vi "UHR-Fleezers Control (host) -TL - oscillation.vi"(0 "Tab Control":T5(tab)) -> ()   [LabVIEW 2013] (continued)
            n1087 = flat-sequence {
              tunnel: w1684 -> [w1698]
              tunnel: w1685 -> [w1694]
              tunnel: w1683 -> [_]
              tunnel: w1685 -> [w1700]
              tunnel: w1684 -> [w1701]
              frame #0 {
                n1088 = local read "All Pump Parameters"() -> (w1693:T6)
                n1089 = Multiply(x=60.0, y="Flush Center Ch Rate (ul/m)") -> (x*y=w1690:dbl)
                n1090 = Unbundle By Name(w1693) -> ("Pump 2"=w1699:T32)
                n1091 = call "Set pump parameters.vi"("Pump write delay (ms)"=w1694, "Volume (uL)"="Flush Center Ch Volume (uL)", "Rate (uL/h)"=w1690, "Units"=3.0, "Pump #"=2.0, "Pump Parameters In"=w1699, "VISA resource name"=w1698) -> ("Pump Parameters Out"=w1692:T32)  [unwired: 3 in]
                n1092 = Bundle By Name(cluster=w1693, "Pump 2"=w1692) -> (w1691:T6)
                n1093 = local write "All Pump Parameters"(w1691) -> ()
                n1094 = Add(x="Flush Center Ch Volume (uL)", y="Total Volume\nFlushed (uL)") -> (x+y=w1687:dbl)
                n1095 = local write "Total Volume\nFlushed (uL)"(w1687) -> ()
              }
              frame #1 {
                n1096 = Wait (ms)(milliseconds to wait=w1700) -> ()  [unwired: 1 out]
              }
              frame #2 {
                n1097 = call "Write to pump.vi"("string"="start", "VISA resource name"=w1701) -> ()  [unwired: 1 out]
              }
            }
            n1098 = local read "Chemyx Syringe Pump Serial Port"() -> (w1684:refnum<visa-resource-name>)
          }
          frame Enabled {
            n1099 = call "hamilton_controller.vi"("Open?"=w1703, "valve"=enum16{"A", "B", "C", "D", "ALL"}."B", "action"=T20."MOVE VALVE") -> ()  [unwired: 8 in, 1 out]
          }
        }
      }
      event "Main:": Value Change {
        n1100 = event-data() -> ()  [unwired: 7 out]
        n1101 = call "hamilton_controller.vi"("Open?"="Main:", "valve"=enum16{"A", "B", "C", "D", "ALL"}."C", "action"=T20."MOVE VALVE") -> ()  [unwired: 8 in, 1 out]
      }
      event "Shunt:": Value Change {
        n1102 = event-data() -> ()  [unwired: 7 out]
        n1103 = call "hamilton_controller.vi"("Open?"="Shunt:", "valve"=enum16{"A", "B", "C", "D", "ALL"}."D", "action"=T20."MOVE VALVE") -> ()  [unwired: 8 in, 1 out]
      }
      event "Flip Green Filter": Value Change {
        n1104 = event-data() -> ()  [unwired: 7 out]
        n1105 = local write "Flip Green Filter"("Flip Green Filter") -> ()
        n1106 = flat-sequence {
          tunnel: w1719 -> [w1724]
          tunnel: w1718 -> [w1723]
          tunnel: [w1721] -> w1716
          tunnel: [w1720] -> w1715
          tunnel: [w1726] -> w1714
          tunnel: w1716 -> [w1726]
          tunnel: [w1725] -> w1713
          tunnel: w1715 -> [w1725]
          tunnel: w1714 -> [w1730]
          tunnel: w1713 -> [w1729]
          tunnel: [w1728] -> w1717
          frame #0 {
            n1107 = xnode "Read/Write Control"("FPGA VI Reference In"=w1724, "error in"=w1723, "Green Filter Flipper"=TRUE) -> ("FPGA VI Reference Out"=w1721:T19, "error out"=w1720:errorcluster)
          }
          frame #1 {
            n1108 = Wait (ms)(milliseconds to wait=u32 100) -> ()  [unwired: 1 out]
          }
          frame #2 {
            n1109 = xnode "Read/Write Control"("FPGA VI Reference In"=w1730, "error in"=w1729, "Green Filter Flipper"=FALSE) -> ("error out"=w1728:errorcluster)  [unwired: 1 out]
          }
        }
      }
      event "Pump 1 contents", "Pump 3 contents": Value Change {
        n1110 = event-data() -> ()  [unwired: 7 out]
        n1111 = local read "Pump 1 contents"() -> (→"Pump 1 cont disp":string)
        n1112 = local read "Pump 3 contents"() -> (→"Pump 3 cont disp":string)
      }
      event "Reset Trap Pos. FB": Value Change {
        n1113 = event-data() -> ()  [unwired: 7 out]
        n1114 = xnode "Read/Write Control"("FPGA VI Reference In"=w1736, "error in"=w1735, "Trap Pos. FB Reset"="Reset Trap Pos. FB") -> ()  [unwired: 2 out]
      }
      event "Trap Pos. FB ON": Value Change {
        n1115 = event-data() -> ()  [unwired: 7 out]
        n1116 = xnode "Read/Write Control"("FPGA VI Reference In"=w1739, "error in"=w1738, "Force feedback"="Trap Pos. FB ON") -> ()  [unwired: 2 out]
      }
      event "Trap Pos. FB Range", "Trap Pos. FB Gains", "Trap Pos. FB Mult Factor", "Trap Pos. FB Offset Factor", "Trap Pos FB Negate Action", "Trap Pos FB Monitor\nT1 or T2": Value Change {
        n1117 = event-data() -> ()  [unwired: 7 out]
        n1118 = xnode "Read/Write Control"("FPGA VI Reference In"=w1748, "error in"=w1747, "Trap Pos. FB Range"="Trap Pos. FB Range", "Trap Pos. FB Gains"="Trap Pos. FB Gains", "Trap Pos. FB Mult Factor"="Trap Pos. FB Mult Factor", "Trap Pos. FB Offset Factor"="Trap Pos. FB Offset Factor", "Trap Pos FB Negate Action"="Trap Pos FB Negate Action", "Trap Pos FB Monitor T1 or T2"="Trap Pos FB Monitor\nT1 or T2", "AI1 X Scale"="Trap Pos. AI1 X Pre-scale") -> ()  [unwired: 2 out]
      }
      event "Trap Pos FB SP": Value Change {
        n1119 = event-data() -> ()  [unwired: 7 out]
        n1120 = xnode "Read/Write Control"("FPGA VI Reference In"=w1751, "error in"=w1750, "Trap Pos. FB SP"="Trap Pos FB SP") -> ()  [unwired: 2 out]
      }
      event "Set SP to Reading": Value Change {
        n1121 = event-data() -> ()  [unwired: 7 out]
        n1122 = local read "Trap Pos FB Monitor\nT1 or T2"() -> (w1759:bool)
        n1123 = local read "Trap X AI1 (DMA)"() -> (w1762:T13)
        n1124 = local read "Trap X (AI1)"() -> (w1765:T1)
        n1125 = Unbundle By Name(w1765) -> ("Trap 1"=w1764:fxp<+/-,16,1>, "Trap 2"=w1763:fxp<+/-,16,1>)
        n1126 = Unbundle By Name(w1762) -> ("Set 1"=w1761:fxp<+/-,16,1>, "Set 2"=w1760:fxp<+/-,16,1>)
        n1127 = Select(t=w1764, s=w1759, f=w1763) -> (s? t:f=w1758:fxp<+/-,16,1>)
        n1128 = Select(t=w1761, s=w1759, f=w1760) -> (s? t:f=w1757:fxp<+/-,16,1>)
        n1129 = Not(x="Set SP Using...") -> (.not. x?=w1752:bool)
        n1130 = Select(t=w1758, s=w1752, f=w1757) -> (s? t:f=w1753:fxp<+/-,16,1>)
        n1131 = xnode "Read/Write Control"("FPGA VI Reference In"=w1755, "error in"=w1754, "Trap Pos. FB SP"=w1753) -> ()  [unwired: 2 out]
        n1132 = local write "Trap Pos FB SP"(w1753) -> ()
      }
      event "Trap Pos. FB Out Scale 2^n": Value Change {
        n1133 = event-data() -> ()  [unwired: 7 out]
        n1134 = Scale By Power Of 2(n="Trap Pos. FB Out Scale 2^n", x=ext 1.0) -> (x*2^n=w1767:ext)
        n1135 = property on="Trap Pos. FB Mult Factor" class="DigNum (strict)"("Val(Sgnl)"=w1767) -> ()  [unwired: 2 in, 2 out]
      }
      event "Trap Pos FB Int Count": Value Change {
        n1136 = event-data() -> ()  [unwired: 7 out]
        n1137 = xnode "Read/Write Control"("FPGA VI Reference In"=w1772, "error in"=w1771, "Trap Pos FB Int Count"="Trap Pos FB Int Count") -> ()  [unwired: 2 out]
      }
    }
    "error out 2" <- w950
    n1138 = node-c288() -> ()  [unwired: 1 in, 1 out]
  }
  n1139 = node-c288() -> (w79:T24)  [unwired: 4 out]
  n1140 = timed-loop "Mouse control: trap position (AOM deflection), set confocal spot from image" {
    tunnel: [w1774] -> w38
    tunnel: w2 -> [w1773]
    timing: w79 -> [_]
    timing-out: [_] -> w78
    stop <- w1774 stop-if-true
    n1141 = node-c288() -> ()  [unwired: 2 out]
    n1142 = event shown="[0] \"Pane\": Mouse Down" {
      selector: _ -> [_ _]
      dyn-events: _ -> [_ _]
      timeout: _ -> [_ _]
      tunnel: w1773 -> [w1777 _]
      event Mouse Down {
        n1143 = event-data() -> ("Time"=w1779:u32, "Coords"=w1778:T8, "Button"=w1780:u16)  [unwired: 6 out]
        n1144 = case shown="1" w1780 {
          tunnel: w1779 -> [_ _ w1883]
          tunnel: w1778 -> [_ w1817 w1881]
          tunnel: w1777 -> [_ _ w1879]
          frame 0, Default {
          }
          frame 1 {
            n1145 = property on="APD 2" class="ImageControl"() -> ("Displayed Image Position"=w1787:cluster{"Left":i32, "Top":i32})  [unwired: 2 in, 2 out]
            n1146 = property on="APD 1" class="ImageControl"() -> ("Displayed Image Position"=w1816:cluster{"Left":i32, "Top":i32})  [unwired: 2 in, 2 out]
            n1147 = property on="Detection Laser X" class="ImageControl"() -> ("Displayed Image Position"=w1813:cluster{"Left":i32, "Top":i32})  [unwired: 2 in, 2 out]
            n1148 = property on="Detection Laser Y" class="ImageControl"() -> ("Displayed Image Position"=w1812:cluster{"Left":i32, "Top":i32})  [unwired: 2 in, 2 out]
            n1149 = property on="APD 2" class="ImageControl"() -> ("Displayed Image Size"=w1786:cluster{"Width":u32, "Height":u32})  [unwired: 2 in, 2 out]
            n1150 = property on="APD 1" class="ImageControl"() -> ("Displayed Image Size"=w1814:cluster{"Width":u32, "Height":u32})  [unwired: 2 in, 2 out]
            n1151 = property on="Detection Laser X" class="ImageControl"() -> ("Displayed Image Size"=w1815:cluster{"Width":u32, "Height":u32})  [unwired: 2 in, 2 out]
            n1152 = property on="Detection Laser Y" class="ImageControl"() -> ("Displayed Image Size"=w1811:cluster{"Width":u32, "Height":u32})  [unwired: 2 in, 2 out]
            n1153 = Unbundle By Name(w1786) -> ("Width"=w1783:u32, "Height"=w1782:u32)
            n1154 = Unbundle By Name(w1787) -> ("Left"=w1785:i32, "Top"=w1784:i32)
            n1155 = Unbundle By Name(w1814) -> ("Width"=w1808:u32, "Height"=w1807:u32)
            n1156 = Unbundle By Name(w1815) -> ("Width"=w1804:u32, "Height"=w1803:u32)
            n1157 = Unbundle By Name(w1811) -> ("Width"=w1800:u32, "Height"=w1799:u32)
            n1158 = Unbundle By Name(w1816) -> ("Left"=w1810:i32, "Top"=w1809:i32)
            n1159 = Unbundle By Name(w1813) -> ("Left"=w1806:i32, "Top"=w1805:i32)
            n1160 = Unbundle By Name(w1812) -> ("Left"=w1802:i32, "Top"=w1801:i32)
            n1161 = Bundle("Left"=w1785, "Top"=w1784, "Width"=w1783, "Height"=w1782) -> (w1781:T33)  [unwired: 1 in]
            n1162 = Bundle("Left"=w1810, "Top"=w1809, "Width"=w1808, "Height"=w1807) -> (w1798:T33)  [unwired: 1 in]
            n1163 = Bundle("Left"=w1806, "Top"=w1805, "Width"=w1804, "Height"=w1803) -> (w1797:T33)  [unwired: 1 in]
            n1164 = Bundle("Left"=w1802, "Top"=w1801, "Width"=w1800, "Height"=w1799) -> (w1796:T33)  [unwired: 1 in]
            n1165 = Build Cluster Array(w1781, w1798, w1797, w1796) -> (w1795:T34)
            n1166 = for {
              tunnel: w1817 -> [w1828]
              tunnel: w1795 -> [w1829] mode=indexing
              shift-right: [w1826] -> w1793
              shift-left: TRUE -> [w1827]
              shift-right: [w1825] -> w1791
              shift-left: _ -> [w1821]
              shift-right: [w1824] -> w1790
              shift-left: _ -> [w1820]
              shift-right: [w1823] -> w1789
              shift-left: _ -> [w1819]
              shift-right: [w1822] -> w1788
              shift-left: _ -> [w1818]
              n1167 = case shown="True" w1827 {
                selector: w1827 -> [w1834 _]
                tunnel: w1829 -> [_ w1843]
                tunnel: w1828 -> [_ w1841]
                tunnel: [w1834 w1839] -> w1826
                tunnel: [w1833 w1838] -> w1825
                tunnel: [w1832 w1837] -> w1824
                tunnel: [w1831 w1836] -> w1823
                tunnel: [w1830 w1835] -> w1822
                tunnel: w1821 -> [w1833 _]
                tunnel: w1820 -> [w1832 _]
                tunnel: w1819 -> [w1831 _]
                tunnel: w1818 -> [w1830 _]
                frame False {
                }
                frame True {
                  n1168 = Unbundle(w1843) -> (w1842:T33)
                  n1169 = call "isclickinwindow.vi"("Image Param"=w1842, "Point32"=w1841) -> ("4 Y"=w1835:i32, "3 Height"=w1836:i32, "2 X"=w1837:i32, "1 Width"=w1838:i32, "In image?"=w1840:bool)  [unwired: 1 in]
                  n1170 = Not(x=w1840) -> (.not. x?=w1839:bool)
                }
              }
            }
            n1171 = Not(x=w1793) -> (.not. x?=w1792:bool)
            n1172 = case shown="True" w1792 {
              tunnel: w1790 -> [_ w1856]
              tunnel: w1788 -> [_ w1855]
              tunnel: w1791 -> [_ w1854]
              tunnel: w1789 -> [_ w1853]
              frame False {
              }
              frame True {
                w1849 = FALSE ("Get Point")
                n1173 = local read "Scan lines (y)"() -> (w1858:u64)
                n1174 = local read "Actual MCL Inc (V)"() -> (w1850:dbl)
                n1175 = local read "Scan steps (MCL)"() -> (w1857:u64)
                n1176 = Divide "Y Pix/step"(x=w1853, y=w1858) -> (x/y=w1865:dbl)
                n1177 = Divide "Y V/pix"(x=w1850, y=w1865) -> (x/y=w1864:dbl)
                n1178 = Divide "Y half step offset"(x=w1850, y=2.0) -> (x/y=w1866:dbl)
                n1179 = Divide "X pix/step"(x=w1854, y=w1857) -> (x/y=w1863:dbl)
                n1180 = Negate(x=w1866) -> (-x=w1867:dbl)
                n1181 = local read "Initial Y"() -> (w1873:dbl)
                n1182 = Multiply(x=w1855, y=w1864) -> (x*y=w1874:dbl)
                n1183 = Divide "X half step offset"(x=w1850, y=2.0) -> (x/y=w1860:dbl)
                n1184 = Divide "X V/pix"(x=w1850, y=w1863) -> (x/y=w1862:dbl)
                n1185 = Multiply(x=w1850, y=w1857) -> (x*y=w1869:dbl)
                n1186 = Compound Arithmetic op=ADD(w1867, w1874, w1873) -> (w1851:dbl)
                "Pointer Y (V)" <- w1851
                n1187 = Multiply(x=w1862, y=w1856) -> (x*y=w1871:dbl)
                n1188 = Negate(x=w1860) -> (-x=w1859:dbl)
                n1189 = local read "Initial X"() -> (w1872:dbl)
                n1190 = Negate(x=w1871) -> (-x=w1870:dbl)
                n1191 = Compound Arithmetic op=ADD(w1859, w1869, w1872, w1870) -> (w1852:dbl)
                "Pointer X (V)" <- w1852
                n1192 = Or(x="Set X Only", y="Set Confocal Spot (X-Y)") -> (x .or. y?=w1845:bool)
                n1193 = Or(x="Set Confocal Spot (X-Y)", y="Set Y Only") -> (x .or. y?=w1844:bool)
                n1194 = case shown="True" w1845 {
                  tunnel: w1852 -> [_ w1875]
                  frame False {
                  }
                  frame True {
                    n1195 = property on="AO2" class="Slide (strict)"("Val(Sgnl)"=w1875) -> ()  [unwired: 2 in, 2 out]
                  }
                }
                n1196 = case shown="True" w1844 {
                  tunnel: w1851 -> [_ w1876]
                  frame False {
                  }
                  frame True {
                    n1197 = property on="AO1" class="Slide (strict)"("Val(Sgnl)"=w1876) -> ()  [unwired: 2 in, 2 out]
                  }
                }
                n1198 = local write "Set Confocal Spot (X-Y)"(w1849) -> ()
                n1199 = local write "Set X Only"(w1849) -> ()
                n1200 = local write "Set Y Only"(w1849) -> ()
              }
            }
          }
          frame 3 {
            n1201 = local read "BD 2 Frequency 1 (MHz)"() -> (w1877:dbl)
            n1202 = local read "BD 1 Frequency 1 (MHz)"() -> (w1878:dbl)
            n1203 = local write "Manipulating Trap"(TRUE ("Manipulating Trap")) -> ()
            n1204 = local write "Coords"(T8 {"Horizontal"=0, "Vertical"=0} ("Coords")) -> ()
            n1205 = while {
              tunnel: w1883 -> [w1888]
              tunnel: w1881 -> [w1887]
              tunnel: w1879 -> [w1886]
              tunnel: w1878 -> [w1885]
              tunnel: w1877 -> [w1884]
              stop <- w1889 stop-if-true
              n1206 = event shown="[0] \"Pane\": Mouse Move" {
                selector: _ -> [_ _]
                dyn-events: _ -> [_ _]
                timeout: _ -> [_ _]
                tunnel: ["Force Manip Abort" w1953] -> w1889
                tunnel: w1888 -> [w1896 _]
                tunnel: w1887 -> [w1894 _]
                tunnel: w1886 -> [w1893 _]
                tunnel: w1885 -> [w1892 _]
                tunnel: w1884 -> [w1891 _]
                event Mouse Move {
                  n1207 = event-data() -> ("Time"=w1897:u32, "Coords"=w1898:T8)  [unwired: 3 out]
                  n1208 = Less?(x=w1897, y=w1896) -> (x < y?=w1895:bool)
                  n1209 = case "Makes sure old motion events prior to mouse click aren't used" shown="False" w1895 {
                    tunnel: w1898 -> [w1940 _]
                    tunnel: w1894 -> [w1941 _]
                    tunnel: w1893 -> [w1918 _]
                    tunnel: w1892 -> [w1914 _]
                    tunnel: w1891 -> [w1913 _]
                    frame False {
                      n1210 = Subtract(x=w1940, y=w1941) -> (x-y=w1939:T8)
                      "Coords" <- w1939
                      n1211 = local read "Y RF Frequency Limits (MHz)"() -> (w1899:T16)
                      n1212 = To Double Precision Float(number=w1939) -> (double precision float=w1938:cluster{"Horizontal":dbl, "Vertical":dbl})
                      n1213 = Multiply(x=cluster{"Horizontal":dbl, "Vertical":dbl} {"Horizontal"=-1.0, "Vertical"=1.0}, y="Manipulation Scaling") -> (x*y=w1934:cluster{"Horizontal":dbl, "Vertical":dbl})
                      n1214 = local read "X RF Frequency Limits (MHz)"() -> (w1900:T16)
                      n1215 = Multiply(x=w1938, y=w1934) -> (x*y=w1936:cluster{"Horizontal":dbl, "Vertical":dbl})
                      n1216 = Unbundle By Name(w1936) -> ("Horizontal"=w1931:dbl, "Vertical"=w1935:dbl)
                      n1217 = Unbundle By Name(w1899) -> ("Maximum"=w1902:dbl, "Minimum"=w1901:dbl)
                      n1218 = Boolean To (0,1)(Boolean="Manip. X?") -> (0, 1=w1929:i16)
                      n1219 = Boolean To (0,1)(Boolean="Manip. Y?") -> (0, 1=w1926:i16)
                      n1220 = local read "BD 1 Frequency 2 (MHz)"() -> (w1916:dbl)
                      n1221 = Multiply(x=w1935, y=w1926) -> (x*y=w1928:dbl)
                      n1222 = Multiply(x=w1929, y=w1931) -> (x*y=w1932:dbl)
                      n1223 = local read "BD 2 Frequency 2 (MHz)"() -> (w1915:dbl)
                      n1224 = Unbundle By Name(w1900) -> ("Maximum"=w1904:dbl, "Minimum"=w1903:dbl)
                      n1225 = Add(x=w1913, y=w1928) -> (x+y=w1906:dbl)
                      n1226 = Add(x=w1914, y=w1932) -> (x+y=w1908:dbl)
                      n1227 = In Range and Coerce(upper limit=w1904, x=w1908, lower limit=w1903) -> (coerced(x)=w1907:dbl)  [unwired: 1 out]
                      n1228 = In Range and Coerce(upper limit=w1902, x=w1906, lower limit=w1901) -> (coerced(x)=w1905:dbl)  [unwired: 1 out]
                      n1229 = Subtract(x=w1907, y=w1916) -> (x-y=w1925:dbl)
                      n1230 = Subtract(x=w1905, y=w1915) -> (x-y=w1924:dbl)
                      n1231 = Square(x=w1925) -> (x^2=w1923:dbl)
                      n1232 = Square(x=w1924) -> (x^2=w1922:dbl)
                      n1233 = Add(x=w1923, y=w1922) -> (x+y=w1921:dbl)
                      n1234 = Square Root(x=w1921) -> (sqrt(x)=w1917:dbl)
                      n1235 = In Range and Coerce(upper limit="Limit Max (MHz)", x=w1917, lower limit="Limit Min (MHz)") -> (In Range?=w1910:bool)  [unwired: 1 out]
                      n1236 = Not(x="Limits Enable") -> (.not. x?=w1909:bool)
                      n1237 = Or(x=w1910, y=w1909) -> (x .or. y?=w1911:bool)
                      n1238 = case shown="True" w1911 {
                        tunnel: w1918 -> [_ w1951]
                        tunnel: w1917 -> [_ w1942]
                        tunnel: w1907 -> [_ w1949]
                        tunnel: w1916 -> [_ w1948]
                        tunnel: w1905 -> [_ w1947]
                        tunnel: w1915 -> [_ w1946]
                        tunnel: w1900 -> [_ w1944]
                        tunnel: w1899 -> [_ w1943]
                        frame False {
                        }
                        frame True {
                          n1239 = local read "BD 1 Frequency 3 (MHz)"() -> (w1950:dbl)
                          n1240 = local read "BD 2 Frequency 3 (MHz)"() -> (w1945:dbl)
                          n1241 = local write "Trap Delta (MHz)"(w1942) -> ()
                          n1242 = property on="Initial delta (MHz)" class="DigNum (strict)"("Val(Sgnl)"=w1942) -> ()  [unwired: 2 in, 2 out]
                          n1243 = call "set RF board frequency - interlace.vi"("Board 2 Frequency Limits"=w1943, "Board 1 Frequency Limits"=w1944, "FPGA VI Reference In"=w1951, "Board 2 Frequency 3 (MHz)"=w1945, "Board 1 Frequency 3 (MHz)"=w1950, "Board 2 Frequency 2 (MHz)"=w1946, "Board 2 Frequency 1 (MHz)"=w1947, "Board 1 Frequency 2 (MHz)"=w1948, "Board 1 Frequency 1  (MHz)"=w1949) -> ()  [unwired: 1 in, 2 out]
                          n1244 = local write "BD 2 Frequency 1 (MHz)"(w1947) -> ()
                          n1245 = local write "BD 1 Frequency 1 (MHz)"(w1949) -> ()
                        }
                      }
                    }
                    frame True {
                    }
                  }
                }
                event Mouse Up {
                  n1246 = event-data() -> ("Button"=w1952:u16)  [unwired: 8 out]
                  n1247 = case shown="3" w1952 {
                    tunnel: [FALSE TRUE] -> w1953
                    frame 0, Default {
                    }
                    frame 3 {
                      n1248 = local write "Manipulating Trap"(FALSE ("Manipulating Trap")) -> ()
                    }
                  }
                }
              }
            }
          }
        }
      }
      event Mouse Move {
        n1249 = event-data() -> ()  [unwired: 6 out]
      }
    }
    n1250 = local read "Stop All"() -> (w1774:bool)
    n1251 = node-c288() -> ()  [unwired: 2 out]
  }
  n1252 = node-c288(w19) -> ()  [unwired: 1 out]
  n1253 = node-c288(w78) -> ()  [unwired: 1 out]
  n1254 = node-c288(w71) -> ()  [unwired: 1 out]
  n1255 = node-c288(i64 1 ("Period"), i64 1 ("Period")) -> (w166:T24)  [unwired: 2 out]
  n1256 = case "Oscillate traps during calibration" shown="True" "Oscillate Traps\n(during calibration)" {
    tunnel: _ -> [_ w1984]
    tunnel: _ -> [_ w1957]
    frame False {
    }
    frame True {
      # "FPGA"
      # "period"
      # "i"
      # "Also note that the 1 ms lower limit per iteration of all LabView loops\nis the reason why the power spectrum shows higher harmonics\nwhen performing a forced oscillation-based calibration procedure.\nOne solution to this would be to implement the osciallation using\nthe FPGA, or to account for the harmonics in the analysis. The forced\noscillation needs to discretized on timescales that won't affect\nthe power spectrum (i.e., > 66 kHz detection bandwidth; < 15 µs)."
      # "Note: Trap Oscillation was originally written\nfor Trap 2!!!  This was modified to oscillation\nboth traps for board 1 (x-axis), but not changed\nfor board 2 (y-axis), since we only implement\nx-axis control at the moment (TL, 1/1/15)"
      n1257 = Wait (ms)(milliseconds to wait=u32 1) -> ()  [unwired: 1 out]
      n1258 = local read "Osc. freq. (Hz)"() -> (w1983:dbl)
      n1259 = Divide(x=i64 1, y=i64 1000) -> (x/y=w1976:dbl)
      n1260 = Multiply(x=w1976, y=w1957) -> (x*y=w1978:dbl)
      n1261 = Multiply(x=w1983, y=6.283185307179586) -> (x*y=w1979:dbl)
      n1262 = Multiply(x=w1979, y=w1978) -> (x*y=w1968:dbl)
      n1263 = local read "BD 1 Frequency 1 (MHz)"() -> (w1960:dbl)
      n1264 = local read "BD 1 Frequency 2 (MHz)"() -> (w1966:dbl)
      n1265 = Sine(x=w1968) -> (sin(x)=w1980:dbl)
      n1266 = local read "Osc. amp. (MHz)"() -> (w1982:dbl)
      n1267 = Multiply(x=w1980, y=w1982) -> (x*y=w1962:dbl)
      n1268 = local read "Scan axis (osc)"() -> (w1981:bool)
      n1269 = Add(x=w1962, y=w1960) -> (x+y=w1963:dbl)
      n1270 = Select(t=w1963, s=w1981, f=w1960) -> (s? t:f=w1961:dbl)
      n1271 = local read "Y RF Frequency Limits (MHz)"() -> (w1970:T16)
      n1272 = local read "X RF Frequency Limits (MHz)"() -> (w1971:T16)
      n1273 = local read "BD 2 Frequency 2 (MHz)"() -> (w1965:dbl)
      n1274 = Select(t=w1966, s=w1981, f=w1965) -> (s? t:f=w1972:dbl)
      n1275 = Add(x=w1962, y=w1972) -> (x+y=w1969:dbl)
      n1276 = Select(t=w1969, s=w1981, f=w1966) -> (s? t:f=w1964:dbl)
      n1277 = Select(t=w1965, s=w1981, f=w1969) -> (s? t:f=w1973:dbl)
      n1278 = local read "BD 2 Frequency 3 (MHz)"() -> (w1974:dbl)
      n1279 = local read "BD 1 Frequency 3 (MHz)"() -> (w1975:dbl)
      n1280 = call "set RF board frequency - interlace.vi"("Board 2 Frequency Limits"=w1970, "Board 1 Frequency Limits"=w1971, "FPGA VI Reference In"=w1984, "Board 2 Frequency 3 (MHz)"=w1974, "Board 1 Frequency 3 (MHz)"=w1975, "Board 2 Frequency 2 (MHz)"=w1965, "Board 2 Frequency 1 (MHz)"=w1973, "Board 1 Frequency 2 (MHz)"=w1964, "Board 1 Frequency 1  (MHz)"=w1961) -> ()  [unwired: 1 in, 2 out]
      "Numeric" <- w1957
    }
  }
  n1281 = timed-loop "Acquire Data" {
    tunnel: w2 -> [w2250]
    tunnel: w44 -> [w2249]
    tunnel: [w2280] -> w37
    tunnel: [w2274] -> w36
    timing: w166 -> [_]
    timing-out: [_] -> w165
    tunnel: w62 -> [w2081]
    stop <- "Stop All" stop-if-true
    (unwired) u32 0 ("Number of Elements")
    w2068 = "NI_ChannelName" ("name")
    n1282 = node-c288() -> ()  [unwired: 2 out]
    n1283 = First Call?() -> (First Call?: T/F=w2034:bool)
    n1284 = Or(x="Reset", y=w2034) -> (x .or. y?=w2035:bool)
    n1285 = case "Reset data stream" shown="True" w2035 {
      tunnel: w2250 -> [w2296 w2304]
      tunnel: w2249 -> [w2295 w2303]
      tunnel: [w2296 w2298] -> w1986
      tunnel: [w2295 w2297] -> w1985
      frame False {
      }
      frame True {
        w2301 = TRUE ("AI to FIFO")
        n1286 = local write "Overflow (data lost)"(FALSE ("Overflow (data lost)")) -> ()
        n1287 = call "reset FPGA DMA.vi"("error in"=w2303, "FPGA VI Reference In"=w2304) -> ("error out"=w2299:errorcluster, "FPGA VI Reference Out"=w2300:T19)
        n1288 = xnode "Read/Write Control"("FPGA VI Reference In"=w2300, "error in"=w2299, "AI to FIFO"=w2301, "APD to FIFO"=w2301) -> ("FPGA VI Reference Out"=w2298:T19, "error out"=w2297:errorcluster)
      }
    }
    n1289 = Or(x="Start AOD Scan", y="Trap Raster Scan") -> (x .or. y?=w2197:bool)
    n1290 = case "Start AOM raster scan" shown="True" w2197 {
      tunnel: w1986 -> [w3033 w3043]
      tunnel: w1985 -> [w3032 w3042]
      tunnel: [w3033 w3036] -> w2245
      tunnel: [w3032 w3035] -> w2244
      frame False {
      }
      frame True {
        n1291 = case shown="True" "Restart DMA? (AOD)" {
          tunnel: [w3081 w3083] -> w3037
          tunnel: [w3080 w3082] -> w3038
          tunnel: w3043 -> [w3081 w3085]
          tunnel: w3042 -> [w3080 w3084]
          frame False {
          }
          frame True {
            n1292 = local write "Overflow (data lost)"(FALSE ("Overflow (data lost)")) -> ()
            n1293 = call "reset FPGA DMA.vi"("error in"=w3084, "FPGA VI Reference In"=w3085) -> ("error out"=w3082:errorcluster, "FPGA VI Reference Out"=w3083:T19)
          }
        }
        n1294 = local write "Trap Raster Scan"(FALSE ("Trap Raster Scan")) -> ()
        n1295 = case shown="True" "Move MCL Also?" {
          tunnel: w3038 -> [w3046 w3075]
          tunnel: w3037 -> [w3047 w3076]
          tunnel: [w3045 w3079] -> w3036
          tunnel: [w3044 w3078] -> w3035
          frame False {
            w3048 = TRUE ("AI to FIFO")
            n1296 = xnode "Read/Write Control"("FPGA VI Reference In"=w3047, "error in"=w3046, "AI to FIFO"=w3048, "APD to FIFO"=w3048, "Start scan"=w3048) -> ("FPGA VI Reference Out"=w3045:T19, "error out"=w3044:errorcluster)
          }
          frame True {
            w3072 = FALSE ("1D or 2D Scan?")
            w3077 = TRUE ("AI to FIFO")
            # "Count for MCL loop"
            # "N total cycles"
            # "N steps"
            # "V_int"
            n1297 = local read "Scan Range (nm)"() -> (w3054:dbl)
            n1298 = local read "Number of F/B Scans (AOD)"() -> (w3071:u16)
            n1299 = Sign(1:w3054) -> (0:w3053:dbl)
            n1300 = Compound Arithmetic op=MULTIPLY(w3054, "MCL Step Position Ratio", "MCL/AOM Scale Tweak") -> (w3058:dbl)
            n1301 = Negate(x=w3053) -> (-x=w3050:dbl)
            n1302 = Multiply(x=w3050, y="MCL Step Increment (V_int)") -> (x*y=w3052:dbl)
            n1303 = Divide(x=w3058, y="MCL X Cal (nm/V)") -> (x/y=w3064:dbl)
            n1304 = Multiply(x=32767.0 ("y"), y=w3064) -> (x*y=w3070:dbl)
            n1305 = local read "Total Counts (ticks)"() -> (w3055:u32)
            n1306 = local read "Cycles/step (AOD)"() -> (w3066:u64)
            n1307 = local read "Scan steps (AOD)"() -> (w3067:u64)
            n1308 = Divide(x=w3070, y=10.0) -> (x/y=w3063:dbl)
            n1309 = Divide(x=w3063, y="MCL Step Increment (V_int)") -> (x/y=w3061:dbl)
            n1310 = Absolute Value(x=w3061) -> (abs(x)=w3049:dbl)
            n1311 = Compound Arithmetic op=MULTIPLY(w3067, w3066, w3055) -> (w3062:u64)
            n1312 = local write "wait to reset values"(w3077) -> ()
            n1313 = local write "MCL Scanning"(w3077) -> ()
            n1314 = Divide(x=w3062, y=w3049) -> (x/y=w3059:dbl)
            "MCL Count" <- w3059
            n1315 = xnode "Read/Write Control"("FPGA VI Reference In"=w3076, "error in"=w3075, "Scan steps (MCL)"=w3049, "Number of scans (MCL)"=w3071, "Cycles per step (MCL)"=u64 1, "Scan freq.  increment (MCL)"=w3052, "1D or 2D Scan?"=w3072, "MCL Scan Axis"=w3072, "Cont. Scan (MCL)"=w3072, "MCL count"=w3059) -> ("FPGA VI Reference Out"=w3074:T19, "error out"=w3073:errorcluster)
            n1316 = xnode "Read/Write Control"("FPGA VI Reference In"=w3074, "error in"=w3073, "AI to FIFO"=w3077, "APD to FIFO"=w3077, "Start scan"=w3077, "Start scan (MCL)"=w3077) -> ("FPGA VI Reference Out"=w3079:T19, "error out"=w3078:errorcluster)
          }
        }
        "Raster Scanning..." <- TRUE ("Scanning...")
      }
    }
    n1317 = And(x="Save scans", y=w2197) -> (x .and. y?=w2243:bool)
    n1318 = Compound Arithmetic op=OR("Start MCL Scan", "Confocal Image", "Confocal Linescan") -> (w2195:bool)
    n1319 = And(x="Save Data (MCL)", y=w2195) -> (x .and. y?=w2242:bool)
    n1320 = case "Start MCL raster scan" shown="True" w2195 {
      tunnel: w2245 -> [w2587 w2602]
      tunnel: w2244 -> [w2586 w2601]
      tunnel: [w2587 w2597] -> w2003
      tunnel: [w2586 w2596] -> w2002
      tunnel: [FALSE w2595] -> w2228
      tunnel: "Start MCL Scan" -> [_ w2590]
      tunnel: "Confocal Image" -> [_ w2589]
      tunnel: "Confocal Linescan" -> [_ _]
      frame False {
      }
      frame True {
        w2595 = TRUE
        n1321 = case shown="True" "Restart DMA? (MCL)" {
          tunnel: [w2647 w2649] -> w2600
          tunnel: [w2646 w2648] -> w2599
          tunnel: w2602 -> [w2647 w2652]
          tunnel: w2601 -> [w2646 w2651]
          frame False {
          }
          frame True {
            n1322 = call "reset FPGA DMA.vi"("error in"=w2651, "FPGA VI Reference In"=w2652) -> ("error out"=w2648:errorcluster, "FPGA VI Reference Out"=w2649:T19)
            n1323 = local write "Overflow (data lost)"(FALSE ("Overflow (data lost)")) -> ()
          }
        }
        n1324 = case shown="False" w2590 {
          selector: w2590 -> [_ w2606]
          tunnel: w2589 -> [w2605 _]
          tunnel: [w2605 w2606] -> w2588
          frame False {
            n1325 = property on="2D or 1D Scan" class="Bool (strict)"("Val(Sgnl)"=w2605) -> ()  [unwired: 2 in, 2 out]
            n1326 = property on="Confocal Image" class="Bool (strict)"("Value"=FALSE ("Start Confocal Map")) -> ()  [unwired: 2 in, 2 out]
          }
          frame True {
          }
        }
        n1327 = local write "MCL Scanning"(w2595) -> ()
        n1328 = local read "AO1"() -> (w2592:dbl)
        n1329 = local read "AO2"() -> (w2591:dbl)
        n1330 = case shown="True" "Center Scan" {
          tunnel: w2600 -> [w2613 w2645]
          tunnel: w2599 -> [w2612 w2644]
          tunnel: [w2611 w2643] -> w2597
          tunnel: [w2610 w2642] -> w2596
          tunnel: [w2608 w2629] -> w2594
          tunnel: [w2607 w2628] -> w2593
          tunnel: w2592 -> [w2608 w2634]
          tunnel: w2591 -> [w2607 w2637]
          tunnel: w2588 -> [_ _]
          frame False {
            w2609 = TRUE ("AI to FIFO")
            n1331 = xnode "Read/Write Control"("FPGA VI Reference In"=w2613, "error in"=w2612, "AI to FIFO"=w2609, "APD to FIFO"=w2609, "Start scan (MCL)"=w2609) -> ("FPGA VI Reference Out"=w2611:T19, "error out"=w2610:errorcluster)
          }
          frame True {
            w2641 = TRUE ("AI to FIFO")
            n1332 = local read "Scan steps (MCL)"() -> (w2620:u64)
            n1333 = local read "Scan lines (y)"() -> (w2616:u64)
            n1334 = local read "Fast Scan Dir"() -> (w2627:bool)
            n1335 = local read "Actual MCL Inc (V)"() -> (w2617:dbl)
            n1336 = Decrement(x=w2616) -> (x-1=w2615:u64)
            n1337 = Decrement(x=w2620) -> (x-1=w2619:u64)
            n1338 = Multiply(x=w2617, y=w2615) -> (x*y=w2614:dbl)
            n1339 = Divide(x=w2614, y=2.0) -> (x/y=w2624:dbl)
            n1340 = Multiply(x=w2617, y=w2619) -> (x*y=w2618:dbl)
            n1341 = Divide(x=w2618, y=2.0) -> (x/y=w2623:dbl)
            n1342 = Select(t=w2623, s=w2627, f=w2624) -> (s? t:f=w2622:dbl)
            n1343 = Select(t=w2624, s=w2627, f=w2623) -> (s? t:f=w2626:dbl)
            n1344 = Subtract(x=w2634, y=w2626) -> (x-y=w2625:dbl)
            n1345 = Subtract(x=w2637, y=w2622) -> (x-y=w2621:dbl)
            n1346 = local read "2D or 1D Scan"() -> (w2639:bool)
            n1347 = Not(x=w2627) -> (.not. x?=w2633:bool)
            n1348 = Not(x=w2639) -> (.not. x?=w2635:bool)
            n1349 = And(x=w2627, y=w2635) -> (x .and. y?=w2636:bool)
            n1350 = And(x=w2635, y=w2633) -> (x .and. y?=w2638:bool)
            n1351 = Select(t=w2637, s=w2638, f=w2621) -> (s? t:f=w2628:dbl)
            n1352 = Select(t=w2634, s=w2636, f=w2625) -> (s? t:f=w2629:dbl)
            n1353 = call "Volt to I16.vi"("Voltage In"=w2629) -> ("I16 Voltage Out"=w2632:i16)
            n1354 = call "Volt to I16.vi"("Voltage In"=w2628) -> ("I16 Voltage Out"=w2631:i16)
            n1355 = xnode "Read/Write Control"("FPGA VI Reference In"=w2645, "error in"=w2644, "AI to FIFO"=w2641, "APD to FIFO"=w2641, "Start scan (MCL)"=w2641, "AO1"=w2632, "AO2"=w2631) -> ("FPGA VI Reference Out"=w2643:T19, "error out"=w2642:errorcluster)
          }
        }
        "Initial Y" <- w2594
        "Initial X" <- w2593
        "wait to reset values" <- w2595
      }
    }
    n1356 = local read "Trap Pos Elements/DMA read"() -> (w2077:u32)
    n1357 = local read "Trap AI Elements/DMA read"() -> (w2001:u32)
    n1358 = local read "APD Elements/DMA read"() -> (w2120:u32)
    n1359 = local read "Trap AI FIFO Depth"() -> (w2290:u32)
    n1360 = xnode "Invoke Method"("FPGA VI Reference In"=w2003, "error in"=w2002, "Number of Elements"=w2077, "Timeout (ms)"=-1) -> ("Data"=w2041:u16[], "Elements Remaining"=→"Trap Pos FIFO El Remaining":u32)  [unwired: 2 out]
    n1361 = xnode "Invoke Method"("FPGA VI Reference In"=w2003, "error in"=w2002, "Number of Elements"=w2001, "Timeout (ms)"=-1 ("Timeout")) -> ("FPGA VI Reference Out"=w2005:T19, "error out"=w2004:errorcluster, "Data"=w2000:i16[], "Elements Remaining"=w2006:u32)
    "Trap AI FIFO El. Rem." <- w2006
    n1362 = xnode "Get APD Data"("FPGA VI Reference In"=w2003, "error in"=w2002, "Number of Elements"=w2120, "Timeout (ms)"=-1) -> ("Data"=w2119:u32[], "Elements Remaining"=→"APD FIFO Elements Remaining":u32)  [unwired: 2 out]
    n1363 = Subtract(x=w2290, y=w2001) -> (x-y=w2289:u32)
    n1364 = Decimate 1D Array(w2041) -> (w2038:u16[], w2040:u16[], w2039:u16[])
    n1365 = Divide(x=w2006, y=w2289) -> (x/y=w2288:dbl)
    "Buffer Status" <- w2288
    n1366 = To Unsigned Long Integer(number=w2038) -> (unsigned 32bit integer=w2037:u32[])
    n1367 = Join Numbers(hi=w2040, lo=w2039) -> ((hi.lo)=w2036:u32[])
    n1368 = Equal?(x=w2288, y=1.0) -> (x = y?=w2286:bool)
    n1369 = Join Numbers(hi=w2037, lo=w2036) -> ((hi.lo)=w2030:u64[])
    n1370 = call "IR AOM word to freq - vec.vi"("Frequency Word In (double vec)"=w2030) -> ("Frequency Out"=w2076:dbl[])
    n1371 = case "Alert buffer overflow" shown="False" w2286 {
      frame False {
      }
      frame True {
        n1372 = call <vilib>:"Beep.vi"() -> ()  [unwired: 3 in, 9 out]
        "Overflow (data lost)" <- TRUE ("Overflow (data lost)")
      }
    }
    n1373 = Decimate 1D Array(w2076) -> (w2075:dbl[], w2074:dbl[])
    n1374 = Array Size(array=w2000) -> (size(s)=→"Waveform Chart":i32)
    n1375 = Build Array(w2075, w2074) -> (w2073:dbl[][])
    n1376 = local read "Trap Sets"() -> (w2157:u32)
    n1377 = case "Deinterlace trap data, average down PSD" shown="2" w2157 {
      tunnel: w2000 -> [w2682 w2747]
      tunnel: [w2679 w2744] -> w2150
      tunnel: [w2682 w2746] -> w2033
      tunnel: "Detector Type" -> [w2681 w2742]
      tunnel: [w2680 w2745] -> w2149
      tunnel: [w2678 w2743] -> w2261
      frame 1, Default {
        n1378 = Divide(x=w2682, y=3276.7) -> (x/y=w2683:dbl[])
        n1379 = Decimate 1D Array(w2683) -> (w2692:dbl[], w2691:dbl[], w2690:dbl[], w2689:dbl[], w2688:dbl[], w2687:dbl[], w2686:dbl[], w2685:dbl[])
        n1380 = case shown="\"IR-QPD + PSD + FB-QPD position\"" w2681 {
          tunnel: w2692 -> [w2716 w2741]
          tunnel: w2691 -> [w2715 w2740]
          tunnel: w2690 -> [w2700 w2718]
          tunnel: w2689 -> [w2701 w2728]
          tunnel: w2688 -> [w2714 w2739]
          tunnel: w2687 -> [w2713 w2738]
          tunnel: w2686 -> [w2697 w2719]
          tunnel: w2685 -> [w2696 w2717]
          tunnel: [w2695 w2725] -> w2680
          tunnel: [w2694 w2724] -> w2679
          tunnel: [w2693 w2723] -> w2678
          frame "IR-QPD + PSD + FB-QPD", Default {
            w2693 = 0  # Channel pattern
            n1381 = Divide(x=w2716, y=w2701) -> (x/y=w2703:dbl[])
            n1382 = Divide(x=w2715, y=w2701) -> (x/y=w2702:dbl[])
            n1383 = Divide(x=w2714, y=w2697) -> (x/y=w2699:dbl[])
            n1384 = Divide(x=w2713, y=w2696) -> (x/y=w2698:dbl[])
            n1385 = Build Array(w2703, w2702, w2701, w2700, w2699, w2698, w2697, w2696) -> (w2694:dbl[][])
            n1386 = Bundle("T1 Y", "T1 X", "T1 Sum", "FB Sum", "PSD Y", "PSD X", "PSD Y Sum", "PSD X Sum") -> (w2712:T41)  [unwired: 1 out]
            n1387 = Cluster To Array(cluster=w2712) -> (array=w2695:string[])
          }
          frame "IR-QPD + PSD + FB-QPD position" {
            w2723 = 3  # Channel pattern
            n1388 = Negate(x=w2719) -> (-x=w2720:dbl[])
            n1389 = Divide(x=w2741, y=w2728) -> (x/y=w2730:dbl[])
            n1390 = Divide(x=w2740, y=w2728) -> (x/y=w2729:dbl[])
            n1391 = Divide(x=w2739, y=w2719) -> (x/y=w2727:dbl[])
            n1392 = Divide(x=w2738, y=w2720) -> (x/y=w2726:dbl[])
            n1393 = Build Array(w2730, w2729, w2728, w2717, w2718, w2727, w2726, w2719) -> (w2724:dbl[][])
            n1394 = Bundle("T1 Y", "T1 X", "T1 Sum", "FB X", "FB Sum", "PSD Y", "PSD X", "PSD Y Sum") -> (w2737:T41)  [unwired: 1 out]
            n1395 = Cluster To Array(cluster=w2737) -> (array=w2725:string[])
          }
        }
      }
      frame 2 {
        n1396 = case shown="\"UCB Fleezers 052511\"" w2742 {
          tunnel: w2747 -> [w2809 w2876 w2904 w3011]
          tunnel: [w2748 w2868 w2899 w2942] -> w2746
          tunnel: [w2775 w2859 w2901 w2989] -> w2745
          tunnel: [w2774 w2823 w2878 w2956] -> w2744
          tunnel: [w2768 w2858 w2941 w2987] -> w2743
          frame "IR-QPD + PSD + FB-QPD", Default {
            w2768 = 1  # Channel pattern
            # "time average x2 the 4th signal and the 4 psd signals (detection laser)"
            # "deinterlace 3 signals from qpd"
            n1397 = Decimate 1D Array(w2809) -> (w2808:i16[], w2807:i16[], w2773:i16[], w2806:i16[], w2796:i16[], w2794:i16[], w2793:i16[], w2791:i16[])
            n1398 = call "downsample 1D array - double.vi"("Ave N"=2.0, "Array In"=w2796) -> ("Array Out"=w2795:dbl[])  [unwired: 1 out]
            n1399 = call "downsample 1D array - double.vi"("Ave N"=2.0, "Array In"=w2791) -> ("Array Out"=w2790:dbl[])  [unwired: 1 out]
            n1400 = call "downsample 1D array - double.vi"("Ave N"=2.0, "Array In"=w2793) -> ("Array Out"=w2792:dbl[])  [unwired: 1 out]
            n1401 = call "downsample 1D array - double.vi"("Ave N"=2.0, "Array In"=w2794) -> ("Array Out"=w2776:dbl[])  [unwired: 1 out]
            n1402 = Decimate 1D Array(w2808) -> (w2805:i16[], w2777:i16[])
            n1403 = Decimate 1D Array(w2807) -> (w2804:i16[], w2802:i16[])
            n1404 = Decimate 1D Array(w2806) -> (w2803:i16[], w2801:i16[])
            n1405 = Decimate 1D Array(w2773) -> (w2772:i16[], w2771:i16[])
            n1406 = Interleave 1D Arrays(w2805, w2804, w2803, w2777, w2802, w2801, w2772, w2771, w2795, w2776, w2792, w2790) -> (w2789:dbl[])
            n1407 = To Word Integer(number=w2789) -> (16bit integer=w2748:i16[])
            n1408 = Divide(x=w2789, y=3276.7) -> (x/y=w2788:dbl[])
            n1409 = Decimate 1D Array(w2788) -> (w2787:dbl[], w2786:dbl[], w2785:dbl[], w2784:dbl[], w2783:dbl[], w2782:dbl[], w2770:dbl[], w2769:dbl[], w2781:dbl[], w2780:dbl[], w2779:dbl[], w2778:dbl[])
            n1410 = Divide(x=w2787, y=w2785) -> (x/y=w2755:dbl[])
            n1411 = Divide(x=w2786, y=w2785) -> (x/y=w2754:dbl[])
            n1412 = Divide(x=w2784, y=w2782) -> (x/y=w2753:dbl[])
            n1413 = Divide(x=w2783, y=w2782) -> (x/y=w2752:dbl[])
            n1414 = Divide(x=w2781, y=w2779) -> (x/y=w2751:dbl[])
            n1415 = Divide(x=w2780, y=w2778) -> (x/y=w2750:dbl[])
            n1416 = Bundle("T1 Y", "T1 X", "T1 Sum", "T2 Y", "T2 X", "T2 Sum", "T1 FB Sum", "T2 FB Sum", "PSD Y", "PSD X", "PSD Y Sum", "PSD X Sum") -> (w2756:T42)  [unwired: 1 out]
            n1417 = Build Array(w2755, w2754, w2785, w2753, w2752, w2782, w2770, w2769, w2751, w2750, w2779, w2778) -> (w2774:dbl[][])
            n1418 = Cluster To Array(cluster=w2756) -> (array=w2775:string[])
          }
          frame "IR-QPD + PSD + FB-QPD X position" {
            w2858 = 2  # Channel pattern
            # "convert\nADC numbers\nto volts"
            # "time average x2 the 3 psd signals (detection laser)"
            # "deinterlace 3 signals from qpds"
            n1419 = Decimate 1D Array(w2876) -> (w2875:i16[], w2874:i16[], w2811:i16[], w2812:i16[], w2821:i16[], w2818:i16[], w2815:i16[], w2846:i16[])
            n1420 = Decimate 1D Array(w2875) -> (w2873:i16[], w2860:i16[])
            n1421 = call "downsample 1D array - I16.vi"("Ave N"=2.0, "Array In"=w2821) -> ("Array Out"=w2819:i16[])  [unwired: 1 in]
            n1422 = call "downsample 1D array - I16.vi"("Ave N"=2.0, "Array In"=w2818) -> ("Array Out"=w2816:i16[])  [unwired: 1 in]
            n1423 = Decimate 1D Array(w2874) -> (w2872:i16[], w2870:i16[])
            n1424 = Decimate 1D Array(w2812) -> (w2871:i16[], w2869:i16[])
            n1425 = Decimate 1D Array(w2846) -> (w2845:i16[], w2843:i16[])
            n1426 = Decimate 1D Array(w2811) -> (w2844:i16[], w2842:i16[])
            n1427 = call "downsample 1D array - I16.vi"("Ave N"=2.0, "Array In"=w2815) -> ("Array Out"=w2813:i16[])  [unwired: 1 in]
            n1428 = Interleave 1D Arrays(w2873, w2872, w2871, w2860, w2870, w2869, w2845, w2844, w2843, w2842, w2819, w2816, w2813) -> (w2868:i16[])
            n1429 = Divide(x=w2868, y=3276.7) -> (x/y=w2867:dbl[])
            n1430 = Decimate 1D Array(w2867) -> (w2866:dbl[], w2865:dbl[], w2864:dbl[], w2863:dbl[], w2862:dbl[], w2861:dbl[], w2834:dbl[], w2832:dbl[], w2831:dbl[], w2829:dbl[], w2828:dbl[], w2827:dbl[], w2824:dbl[])
            n1431 = Divide(x=w2866, y=w2864) -> (x/y=w2850:dbl[])
            n1432 = Divide(x=w2865, y=w2864) -> (x/y=w2849:dbl[])
            n1433 = Divide(x=w2863, y=w2861) -> (x/y=w2848:dbl[])
            n1434 = Divide(x=w2862, y=w2861) -> (x/y=w2847:dbl[])
            n1435 = Divide(x=w2834, y=w2832) -> (x/y=w2833:dbl[])
            n1436 = Divide(x=w2831, y=w2829) -> (x/y=w2830:dbl[])
            n1437 = Divide(x=w2828, y=w2824) -> (x/y=w2826:dbl[])
            n1438 = Negate(x=w2824) -> (-x=w2822:dbl[])
            n1439 = Divide(x=w2827, y=w2822) -> (x/y=w2825:dbl[])
            n1440 = Bundle("T1 Y", "T1 X", "T1 Sum", "T2 Y", "T2 X", "T2 Sum", "T1 FB X", "T1 FB Sum", "T2 FB X", "T2 FB Sum", "PSD Y", "PSD X", "PSD Y Sum") -> (w2851:T43)  [unwired: 1 out]
            n1441 = Build Array(w2850, w2849, w2864, w2848, w2847, w2861, w2833, w2832, w2830, w2829, w2826, w2825, w2824) -> (w2823:dbl[][])
            n1442 = Cluster To Array(cluster=w2851) -> (array=w2859:string[])
          }
          frame "UCB Fleezers 052511" {
            w2941 = 2  # Channel pattern
            n1443 = Decimate 1D Array(w2904) -> (w2939:i16[], w2938:i16[], w2903:i16[], w2902:i16[], w2896:i16[], w2893:i16[], w2892:i16[], w2891:i16[])
            n1444 = Decimate 1D Array(w2939) -> (w2937:i16[], w2922:i16[])
            n1445 = Decimate 1D Array(w2938) -> (w2936:i16[], w2934:i16[])
            n1446 = Decimate 1D Array(w2903) -> (w2935:i16[], w2933:i16[])
            n1447 = Decimate 1D Array(w2902) -> (w2898:i16[], w2897:i16[])
            n1448 = Decimate 1D Array(w2896) -> (w2895:i16[], w2894:i16[])
            n1449 = call "downsample 1D array - I16.vi"("Ave N"=2.0, "Array In"=w2893) -> ("Array Out"=w2890:i16[])  [unwired: 1 in]
            n1450 = call "downsample 1D array - I16.vi"("Ave N"=2.0, "Array In"=w2892) -> ("Array Out"=w2889:i16[])  [unwired: 1 in]
            n1451 = call "downsample 1D array - I16.vi"("Ave N"=2.0, "Array In"=w2891) -> ("Array Out"=w2888:i16[])  [unwired: 1 in]
            n1452 = Interleave 1D Arrays(w2937, w2936, w2935, w2922, w2934, w2933, w2898, w2895, w2897, w2894, w2890, w2889, w2888) -> (w2899:i16[])
            n1453 = Divide(x=w2899, y=3276.7) -> (x/y=w2929:dbl[])
            n1454 = Decimate 1D Array(w2929) -> (w2928:dbl[], w2927:dbl[], w2926:dbl[], w2925:dbl[], w2924:dbl[], w2923:dbl[], w2887:dbl[], w2885:dbl[], w2884:dbl[], w2882:dbl[], w2881:dbl[], w2880:dbl[], w2879:dbl[])
            n1455 = Divide(x=w2928, y=w2926) -> (x/y=w2909:dbl[])
            n1456 = Divide(x=w2927, y=w2926) -> (x/y=w2908:dbl[])
            n1457 = Divide(x=w2925, y=w2923) -> (x/y=w2907:dbl[])
            n1458 = Divide(x=w2924, y=w2923) -> (x/y=w2906:dbl[])
            n1459 = Divide(x=w2887, y=w2885) -> (x/y=w2886:dbl[])
            n1460 = Divide(x=w2884, y=w2882) -> (x/y=w2883:dbl[])
            n1461 = Bundle("T1 Y", "T1 X", "T1 Sum", "T2 Y", "T2 X", "T2 Sum", "T1 FB X", "T2 FB Sum", "T2 FB X", "T2 FB Sum", "PSD Y", "PSD X", "PSD Sum") -> (w2910:T43)  [unwired: 1 out]
            n1462 = Build Array(w2909, w2908, w2926, w2907, w2906, w2923, w2886, w2885, w2883, w2882, w2881, w2880, w2879) -> (w2878:dbl[][])
            n1463 = Cluster To Array(cluster=w2910) -> (array=w2901:string[])
          }
          frame "IR-QPD + PSD + FB-QPD XY positions" {
            w2987 = 4  # Channel pattern
            # "time average x2 the 3 psd signals (detection laser)"
            # "deinterlace 3 signals from qpds"
            n1464 = Decimate 1D Array(w3011) -> (w3010:i16[], w3009:i16[], w2988:i16[], w3008:i16[], w2954:i16[], w3000:i16[], w2999:i16[], w2976:i16[])
            n1465 = Decimate 1D Array "QPD Y"(w3010) -> (w3007:i16[], w2990:i16[])
            n1466 = call "downsample 1D array - double.vi"("Ave N"=2.0, "Array In"=w3000) -> ("Array Out"=w2975:dbl[])  [unwired: 1 out]
            n1467 = call "downsample 1D array - double.vi"("Ave N"=2.0, "Array In"=w2999) -> ("Array Out"=w2974:dbl[])  [unwired: 1 out]
            n1468 = Decimate 1D Array "Feedback Sum"(w2988) -> (w2972:i16[], w2970:i16[])
            n1469 = Decimate 1D Array "Feedback Y"(w2954) -> (w2953:i16[], w2952:i16[])
            n1470 = Decimate 1D Array "Feedback X"(w2976) -> (w2973:i16[], w2971:i16[])
            n1471 = Decimate 1D Array "QPD Sum"(w3008) -> (w3005:i16[], w3003:i16[])
            n1472 = Decimate 1D Array "QPD X"(w3009) -> (w3006:i16[], w3004:i16[])
            n1473 = Interleave 1D Arrays(w3007, w3006, w3005, w2990, w3004, w3003, w2953, w2973, w2972, w2952, w2971, w2970, w2975, w2974) -> (w2998:dbl[])
            n1474 = To Word Integer(number=w2998) -> (16bit integer=w2942:i16[])
            n1475 = Divide(x=w2998, y=3276.7) -> (x/y=w2997:dbl[])
            n1476 = Decimate 1D Array(w2997) -> (w2996:dbl[], w2995:dbl[], w2994:dbl[], w2993:dbl[], w2992:dbl[], w2991:dbl[], w2949:dbl[], w2963:dbl[], w2947:dbl[], w2948:dbl[], w2961:dbl[], w2945:dbl[], w2959:dbl[], w2957:dbl[])
            n1477 = Divide(x=w2996, y=w2994) -> (x/y=w2980:dbl[])
            n1478 = Divide(x=w2995, y=w2994) -> (x/y=w2979:dbl[])
            n1479 = Divide(x=w2993, y=w2991) -> (x/y=w2978:dbl[])
            n1480 = Divide(x=w2992, y=w2991) -> (x/y=w2977:dbl[])
            n1481 = Divide(x=w2949, y=w2947) -> (x/y=w2946:dbl[])
            n1482 = Divide(x=w2963, y=w2947) -> (x/y=w2962:dbl[])
            n1483 = Divide(x=w2948, y=w2945) -> (x/y=w2944:dbl[])
            n1484 = Divide(x=w2961, y=w2945) -> (x/y=w2960:dbl[])
            n1485 = Negate(x=w2957) -> (-x=w2955:dbl[])
            n1486 = Divide(x=w2959, y=w2955) -> (x/y=w2958:dbl[])
            n1487 = Bundle("T1 Y", "T1 X", "T1 Sum", "T2 Y", "T2 X", "T2 Sum", "T1 FB Y", "T1 FB X", "T1 FB Sum", "T2 FB Y", "T2 FB X", "T2 FB Sum", "PSD X", "PSD Y Sum") -> (w2943:T44)  [unwired: 1 out]
            n1488 = Build Array(w2980, w2979, w2994, w2978, w2977, w2991, w2946, w2962, w2947, w2944, w2960, w2945, w2958, w2957) -> (w2956:dbl[][])
            n1489 = Cluster To Array(cluster=w2943) -> (array=w2989:string[])
          }
        }
      }
    }
    "AI labels" <- w2149
    n1490 = Decimate 1D Array(w2119) -> (w2147:u32[], w2083:u32[])
    n1491 = local read "DMA Update Period (s)"() -> (w2158:dbl)
    n1492 = local read "BD 1 Frequency 2 (MHz)"() -> (w2025:dbl)
    n1493 = local read "BD 1 Frequency 1 (MHz)"() -> (w2026:dbl)
    n1494 = Build Array(w2147, w2083) -> (w2225:u32[][])
    n1495 = local read "Data Period (s)"() -> (w2132:dbl)
    n1496 = Decimate 1D Array(w2033) -> (w2056:i16[], w2055:i16[], w2053:i16[], w2052:i16[])  [unwired: 9 out]
    n1497 = To Double Precision Float(number=w2225) -> (double precision float=w2226:dbl[][])
    n1498 = local read "APD Integration Time (s)"() -> (w2096:dbl)
    n1499 = Divide(x=w2056, y=w2055) -> (x/y=w2057:dbl[])
    n1500 = Divide(x=w2053, y=w2052) -> (x/y=w2054:dbl[])
    n1501 = feedback #1(0.0) -> (w2070:dbl)
    n1502 = Add(x=w2158, y=w2070) -> (x+y=w2263:dbl)
    n1503 = feedback-in #1(w2263) -> ()
    n1504 = local read "AOM X Cal (nm/MHz)"() -> (w2023:dbl)
    n1505 = To Time Stamp(1:w2070) -> (0:w2069:timestamp)
